vi "Trigger.vi"(8 "error in (no error)":errorcluster, 11 "DAQmx Digitizer in":refnum<class "DAQmx Digitizer.lvclass">) -> (0 "error out":errorcluster, 3 "DAQmx Digitizer out":refnum<class "DAQmx Digitizer.lvclass">)   [LabVIEW 2021, in "DAQmx Digitizer.lvclass"]
uses:
  DAQmx Digitizer.lvclass
  DAQmx Digitizer.lvclass/DAQmx Digitizer.ctl
  <vilib>/DAQmx/configure/trigger.llb/DAQmx Reference Trigger (None).vi
  <vilib>/DAQmx/configure/trigger.llb/DAQmx Start Trigger (None).vi
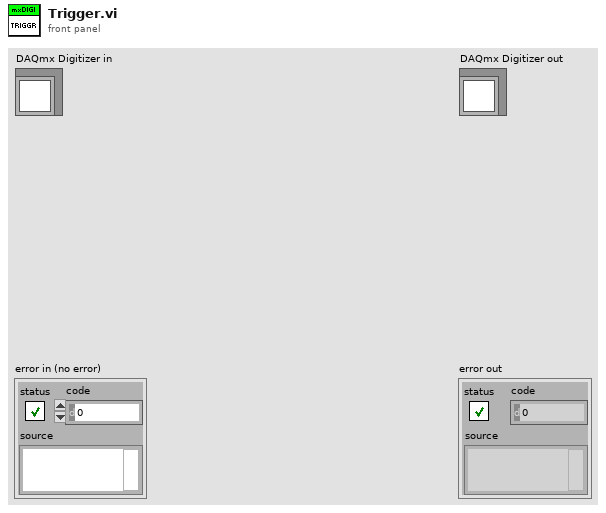
[diagram p1: front panel]
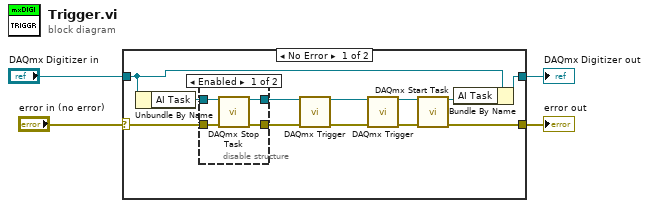
[diagram p0: block diagram]
diagram:
  n1 = case shown="No Error" "error in (no error)" {
    selector: "error in (no error)" -> [w15 w23]
    tunnel: "DAQmx Digitizer in" -> [w12 w24]
    tunnel: [w10 w23] -> w2
    tunnel: [w9 w24] -> w1
    frame No Error {
      n2 = Unbundle By Name(w12) -> ("AI Task"=w16:refnum<k21>)
      n3 = disable-structure shown="Enabled" {
        disable-tunnel: w16 -> [w20 w21]
        disable-tunnel: w15 -> [w19 w22]
        disable-tunnel: [w18 w21] -> w14
        disable-tunnel: [w17 w22] -> w13
        frame Enabled {
          n4 = call <vilib>:"DAQmx Stop Task.vi"("task/channels in"=w20, "error in"=w19) -> ("task out"=w18:refnum<k21>, "error out"=w17:errorcluster)  [unwired: 12 in]
        }
        frame Disabled {
        }
      }
      n5 = call-poly <vilib>:"DAQmx Trigger.vi"("task/channels in"=w14, "error in"=w13) -> ("task out"=w6:refnum<k21>, "error out"=w8:errorcluster)  [unwired: 12 in]
      n6 = call-poly <vilib>:"DAQmx Trigger.vi"("task/channels in"=w6, "error in"=w8) -> ("task out"=w5:refnum<k21>, "error out"=w7:errorcluster)  [unwired: 12 in]
      n7 = call <vilib>:"DAQmx Start Task.vi"("task/channels in"=w5, "error in"=w7) -> ("task out"=w11:refnum<k21>, "error out"=w10:errorcluster)  [unwired: 12 in]
      n8 = Bundle By Name(cluster=w12, "AI Task"=w11) -> (w9:refnum<class "DAQmx Digitizer.lvclass">)
    }
    frame Error {
    }
  }
  "error out" <- w2
  "DAQmx Digitizer out" <- w1
